vi "DMM RM Resistance 2W_4W Individual.vi"() -> ()   [LabVIEW 2021]
uses:
  DMM_Resistance Measurement/DMM Resistance Typedefs/Function Settings.ctl
  <instrlib>/niDMM/nidmm.llb/niDMM Resolution in Digits.ctl
  DMM_Resistance Measurement/DMM Resistance Typedefs/Timing & Trigger Settings.ctl
  <instrlib>/niDMM/nidmm.llb/niDMM Trigger.ctl
  <instrlib>/niDMM/nidmm.llb/niDMM Slope.ctl
  DMM_Resistance Measurement/DMM Resistance Typedefs/Measurement.ctl
  DMM_Resistance Measurement/DMM Resistance Typedefs/DMM Execution Settings.ctl
  <instrlib>/niDMM/nidmm.llb/niDMM Powerline Frequency.ctl
  DMM_Resistance Measurement/DMM_Resistance Measurement.lvlib
panel:
  in  "error in":errorcluster
  in  "Powerline Frequency":T1=enum."50 Hz"
  in  "DMM Resource Name":refnum<k15>="DMM_4080"
  out "DMM Execution Settings":T2={"Absolute\nResolution"=0.004999999999999999, "Input Resistance\n(Ohm)"=0.0, "Digits\nResolution"=6.5, "Range"=10000.0, "Minimum\nFrequency (Hz)"=20.0, "Aperture\nTime (s)"=0.1, "Auto Range\nValue"=10000.0, "Settle\nTime (s)"=0.005, "Function"=5} {"Function" items=["DC Volts"=1, "AC Volts"=2, "DC Current"=3, "AC Current"=4, "2-Wire Resistance"=5, "4-Wire Resistance"=101, "Frequency"=104, "Period"=105, "AC Volts DC Coupled"=1001, "Diode"=1002, "Waveform Voltage"=1003, "Waveform Current"=1004, "Capacitance"=1005, "Inductance"=1006, "Temperature"=108]; "Absolute\nResolution" format="%#_6p"; "Input Resistance\n(Ohm)" format="%#_6p"; "Range" format="%#_6p"; "Minimum\nFrequency (Hz)" format="%#_6p"; "Aperture\nTime (s)" format="%#_6p"; "Auto Range\nValue" format="%#_6p"; "Settle\nTime (s)" format="%#_6p"}
  out "Measurement":T3={"Measured Value"=9879.136917300453, "Out of Range"=FALSE, "Unit"="Ohm", "Measurement"="9.879137kOhm"} {"Measured Value" format="%^#_9e"}
  in  "Timing and Trigger Settings":T4={"Aperture Time (s)"=-1.0, "Settle Time (s)"=-1.0, "Trigger Settings"={"Trigger Delay (sec)"=-1.0, "Enable Trigger?"=FALSE, "Trigger Source"=enum."Immediate", "Slope"=enum."Rising Edge"}} {"Trigger Settings"."Trigger Delay (sec)" format="%.4f"; "Aperture Time (s)" format="%#.6g"}
  in  "Function Settings":T7={"Range and Function"=enum."2w-Res 10 kOhm", "Resolution in Digits"=6.5} {"Resolution in Digits" items=["3 1/2"=3.5, "4 1/2"=4.5, "5 1/2"=5.5, "6 1/2"=6.5, "7 1/2"=7.5]}
  out "error out":errorcluster
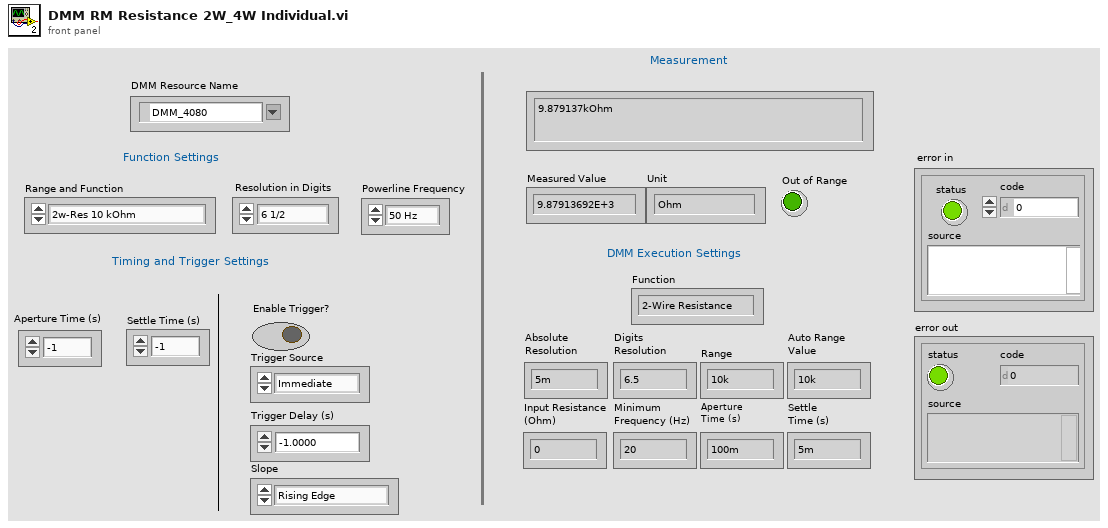
[diagram p1: front panel]
types:
  T1 = typedef "niDMM Powerline Frequency.ctl" = enum16{"60 Hz", "50 Hz"}
  T2 = typedef "DMM_Resistance Measurement.lvlib/DMM Execution Settings.ctl" = cluster{"Absolute\nResolution":dbl, "Input Resistance\n(Ohm)":dbl, "Digits\nResolution":dbl, "Range":dbl, "Minimum\nFrequency (Hz)":dbl, "Aperture\nTime (s)":dbl, "Auto Range\nValue":dbl, "Settle\nTime (s)":dbl, "Function":i32}
  T3 = typedef "DMM_Resistance Measurement.lvlib/Measurement.ctl" = cluster{"Measured Value":dbl, "Out of Range":bool, "Unit":string, "Measurement":string}
  T4 = typedef "DMM_Resistance Measurement.lvlib/Timing & Trigger Settings.ctl" = cluster{"Aperture Time (s)":dbl, "Settle Time (s)":dbl, "Trigger Settings":cluster{"Trigger Delay (sec)":dbl, "Enable Trigger?":bool, "Trigger Source":T5, "Slope":T6}}
  T5 = typedef "niDMM Trigger.ctl" = enum16{"Immediate", "External", "TTL 0", "TTL 1", "TTL 2", "TTL 3", "TTL 4", "TTL 5", "TTL 6", "Software", "TTL 7", "PXI Star", "LBR Trig 1", "Aux Trig 1"}
  T6 = typedef "niDMM Slope.ctl" = enum16{"Rising Edge", "Falling Edge"}
  T7 = typedef "DMM_Resistance Measurement.lvlib/Function Settings.ctl" = cluster{"Range and Function":enum16{"2w-Resistance Auto Range", "2w-Res 100 Ohm", "2w-Res 1 kOhm", "2w-Res 10 kOhm", "2w-Res 100 kOhm", "2w-Res 1 MOhm", "2w-Res 10 MOhm", "2w-Res 100 MOhm", "2w-Res 5 GOhm", "     ", "4w-Resistance Auto Range", "4w-Res 100 Ohm", "4w-Res 1 kOhm", "4w-Res 10 kOhm", "4w-Res 100 kOhm", "4w-Res 1 MOhm", "4w-Res 10 MOhm"}, "Resolution in Digits":T8}
  T8 = typedef "niDMM Resolution in Digits.ctl" = dbl
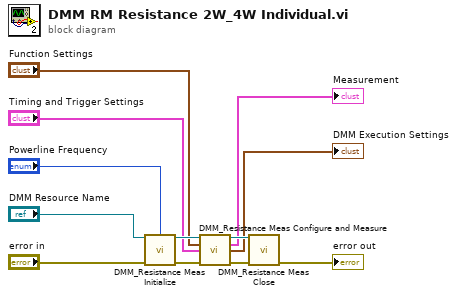
[diagram p0: block diagram]
diagram:
  n1 = call "DMM_Resistance Meas Initialize.vi"("DMM Resource Name"="DMM Resource Name", "Powerline Frequency"="Powerline Frequency", "error in"="error in") -> ("DMM Handle Out"=w12:refnum<k15>, "error out"=w11:errorcluster)  [unwired: 11 in]
  n2 = call "DMM_Resistance Meas Configure and Measure.vi"("DMM Handle In"=w12, "Function Settings"="Function Settings", "Timing and Trigger Settings"="Timing and Trigger Settings", "error in"=w11) -> ("DMM Handle Out"=w10:refnum<k15>, "Measurement"=→"Measurement":T3, "DMM Execution Settings"=→"DMM Execution Settings":T2, "error out"=w9:errorcluster)  [unwired: 8 in]
  n3 = call "DMM_Resistance Meas Close.vi"("DMM Handle In"=w10, "error in"=w9) -> ("error out"=→"error out":errorcluster)  [unwired: 13 in]
